vi "String Array to CSV text.vi"(7 "String_Array":string[][](array[string])) -> (8 "CSV_text":string)   [LabVIEW 2013]
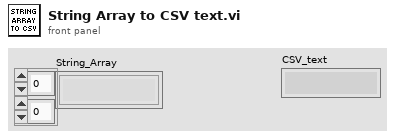
[diagram p1: front panel]
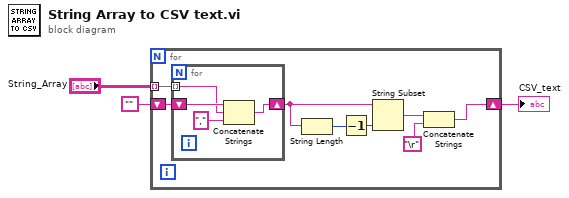
[diagram p0: block diagram]
diagram:
  n1 = for {
    tunnel: "String_Array" -> [w11] mode=indexing
    shift-right: [w4] -> w1
    shift-left: "" -> [w10]
    n2 = for {
      tunnel: w11 -> [w14] mode=indexing
      shift-right: [w12] -> w9
      shift-left: w10 -> [w15]
      n3 = Concatenate Strings(w15, w14, ",") -> (w12:string)
    }
    n4 = String Length(string=w9) -> (length=w8:i32)
    n5 = Decrement(x=w8) -> (x-1=w7:i32)
    n6 = String Subset(string=w9, length (rest)=w7) -> (substring=w6:string)  [unwired: 1 in]
    n7 = Concatenate Strings(w6, "\r") -> (w4:string)
  }
  "CSV_text" <- w1
